vi "struct_ads_sur_T_pwpsat.vi"(7 "Saturation vapor pressure in Pa (Input)":dbl, 8 "Error (Input)":errorcluster, 9 "Loading in kg/kg (Input)":dbl, 10 "Pressure in Pa (Input)":dbl, 11 "Reference working pair (Input)":i64) -> (0 "Error (Output)":errorcluster caption="Error(Output)", 3 "Equilibrium temperature in K (Output)":dbl)   [LabVIEW 2017]
doc: "ads_sur_T_pwpsat:\n * -----------------\n *\n * Calculates equilibrium temperature in K depending on equilibrium pressure p\n * in Pa, equilibrium loading w in kg/kg, and saturation pressure p_sat in Pa.\n *\n * Parameters:\n * -----------\n * double p_Pa:\n * Equilibrium pressure in Pa.\n * double w_kgkg:\n * Equilibrium loading in kg/kg.\n * double p_sat_Pa:\n * Saturation vapor pressure in Pa.\n * struct *WorkingPair:\n * Pointer of WorkingPair-struct.\n *\n * Returns:\n * --------\n * double:\n * Equilibrium temperature in K.\n *\n * Remarks:\n * --------\n * This function is only valid for isotherm models based on the surface\n * approach using the saturated vapor pressure as additional argument.\n * Uses internal equation of states to calculate vapor pressure and derivative\n * of vapor pressure wrt. temperature. If equation of state is not implemented\n * for refrigerant, function returns -1 and throws warning. If user want to use\n * his own equation of state, this function cannot be used and determination of\n * root to calculate T must be implemented by user.\n *\n * History:\n * --------\n * 07/13/2021, by Jannik Driesel (supervised by Mirko Engelpracht):\n * First implementation."
uses:
  data/win32bit/libsorpPropLib.dll
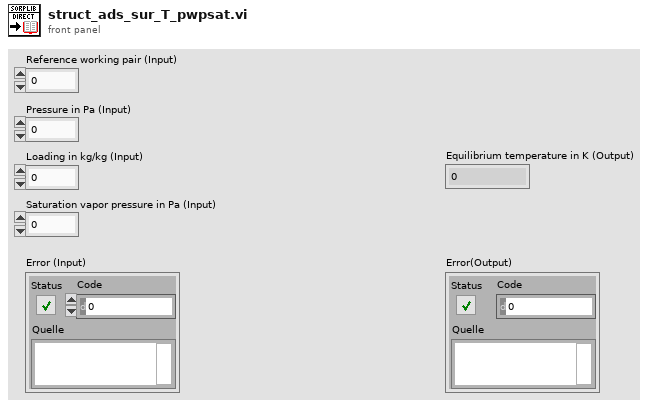
[diagram p1: front panel]
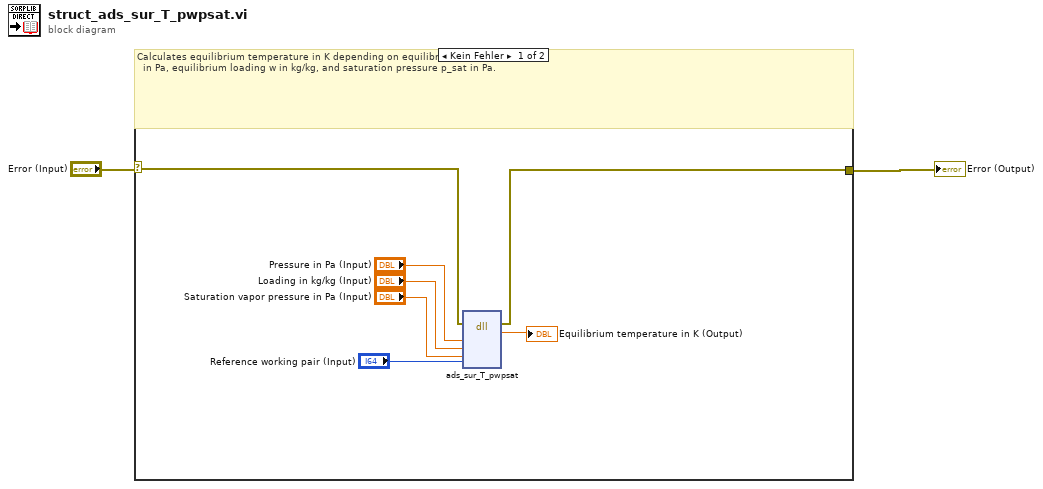
[diagram p0: block diagram]
diagram:
  n1 = case shown="Kein Fehler" "Error (Input)" {
    selector: "Error (Input)" -> [w8 w10]
    tunnel: [w7 w10] -> w1
    frame No Error {
      # "Calculates equilibrium temperature in K depending on equilibrium pressure p\n  in Pa, equilibrium loading w in kg/kg, and saturation pressure p_sat in Pa."
      n2 = dll-call lib="D:/Driesel/SorpLibLocal/LabVIEW_wrapper/data/win32bit/libsorpPropLib.dll" fn="ads_sur_T_pwpsat"(error in=w8, "p_Pa"="Pressure in Pa (Input)", "w_kgkg"="Loading in kg/kg (Input)", "p_sat_pa"="Saturation vapor pressure in Pa (Input)", "workingPair"="Reference working pair (Input)") -> (error out=w7:errorcluster, "T_K"=→"Equilibrium temperature in K (Output)":dbl)  [unwired: 6 in, 1 out]
    }
    frame Error {
      # "Error - No calculations"
    }
  }
  "Error (Output)" <- w1
